vi "Logging Message Loop.vi"(6 "Metadata All":T1={"Data Fields"={"operatorName"="", "project"="", "measurementType"="", "sphere"="", "spectrometer"="", "powerSource"="", "analyzer"="", "fixtureType"="", "lampType"="", "sourceType"="", "testOrientation"="", "model"="", "sample"="", "hours"=".csv", "Amp Gain Range"=""}, "Metadata Disable"={"spectrometer"=enum."Disabled and Grayed Out", "sphere"=enum."Disabled and Grayed Out", "analyzer"=enum."Disabled and Grayed Out", "ampGainRange"=enum."Disabled and Grayed Out"}, "Output Path"=path "C:/Users/dhstuart/Dropbox/CLTC/YokogawaPZ4000/Output"}, 8 "error in (no error)":errorcluster, 9 "Stand alone?":bool=TRUE, 10 "Data Queue":refnum<queue>, 11 "Message Queues":T4) -> (0 "error out":errorcluster)   [LabVIEW 2013, in "Cal Inst Logging.lvlib"]
doc: "The message loop subVI to handle messages pertaining to logging data."
uses:
  Cal Inst Logging.lvlib
  support/Message Queue/All Message Queues.ctl
  support/Message Queue/Message Cluster.ctl
  controls/electrical2.ctl
  controls/Metadata all typedef.ctl
  controls/Metadata typedef.ctl
  controls/Metadata disable typedef.ctl
  Settings/Settings.ctl
  Acquisition/Hardware Configuration.ctl
  Logging Configuration.ctl
  Logging State.ctl
  <vilib>/Utility/error.llb/Error Cluster From Error Code.vi
  <vilib>/ErrorRing/Error Ring.xnode
  support/Message Queue/Cal Inst Message Queue.lvlib
  Acquisition/Cal Inst Acquisition.lvlib
  Settings/Cal Inst Settings.lvlib
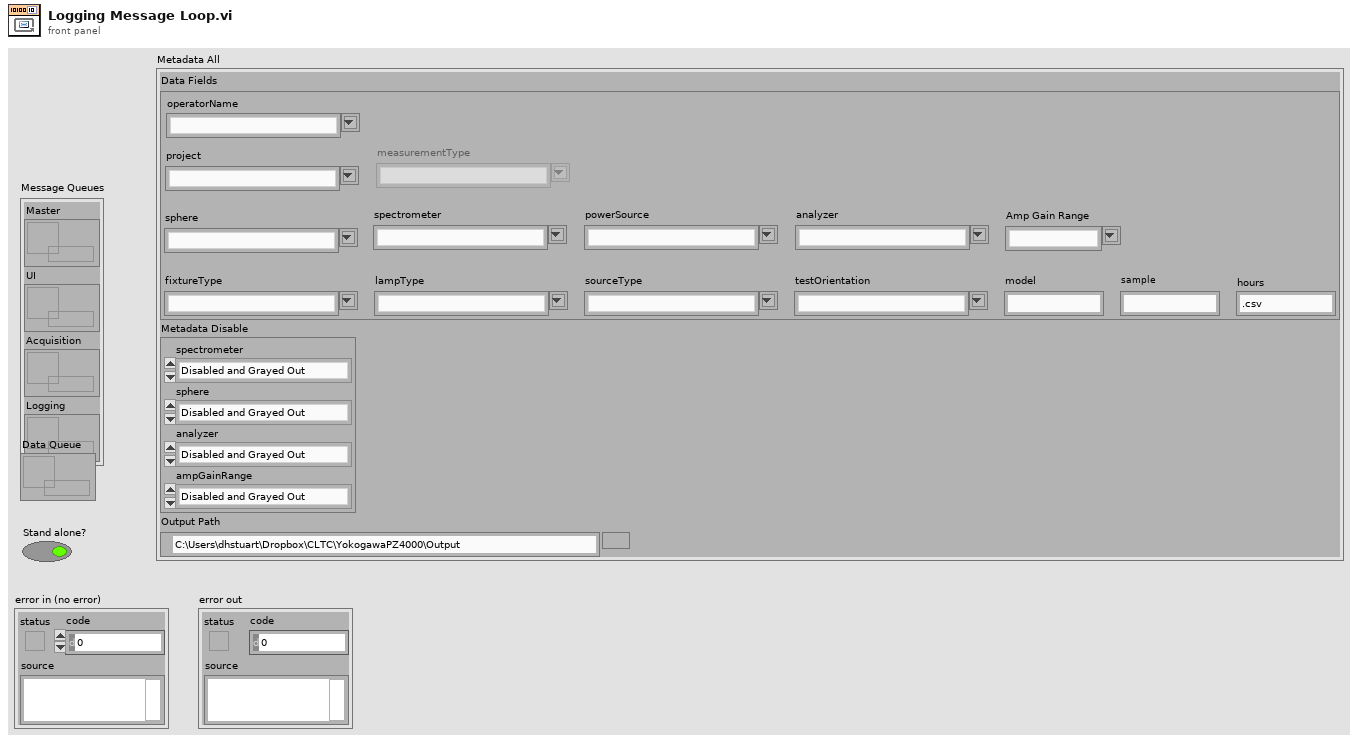
[diagram p1: front panel]
types:
  T1 = typedef "Cal Inst Logging.lvlib/Metadata all typedef.ctl" = cluster{"Data Fields":T2, "Metadata Disable":T3, "Output Path":path}
  T2 = typedef "Cal Inst Logging.lvlib/Metadata typedef.ctl" = cluster{"operatorName":string, "project":string, "measurementType":string, "sphere":string, "spectrometer":string, "powerSource":string, "analyzer":string, "fixtureType":string, "lampType":string, "sourceType":string, "testOrientation":string, "model":string, "sample":string, "hours":string, "Amp Gain Range":string}
  T3 = typedef "Cal Inst Logging.lvlib/Metadata disable typedef.ctl" = cluster{"spectrometer":enum8{"Enabled", "Disabled", "Disabled and Grayed Out"}, "sphere":enum8{"Enabled", "Disabled", "Disabled and Grayed Out"}, "analyzer":enum8{"Enabled", "Disabled", "Disabled and Grayed Out"}, "ampGainRange":enum8{"Enabled", "Disabled", "Disabled and Grayed Out"}}
  T4 = typedef "Cal Inst Message Queue.lvlib/All Message Queues.ctl" = cluster{"Master":refnum<queue>, "UI":refnum<queue>, "Acquisition":refnum<queue>, "Logging":refnum<queue>}
  T5 = typedef "Cal Inst Settings.lvlib/Settings.ctl" = cluster{"Hardware Configuration":T6, "Logging Configuration":T7}
  T6 = typedef "Cal Inst Acquisition.lvlib/Hardware Configuration.ctl" = cluster{"VISA Refnum in":refnum<visa-resource-name>, "Serial Configuration":cluster{"Baud Rate":u32, "Flow Control":u16}, "Voltage Level (0V)":dbl, "Output Phase(s) (1-Phase)":u16, "Active Phase (1:Phase 1)":i32}
  T7 = typedef "Cal Inst Logging.lvlib/Logging Configuration.ctl" = cluster{"Log File Base Path":path, "TDMS File Reference":refnum<k34>}
  T8 = typedef "Cal Inst Logging.lvlib/Logging State.ctl" = enum16{"Idle", "Logging"}
  T9 = enum16{"open", "open or create", "create or replace", "create", "open (read-only)"}
  T10 = typedef "Cal Inst Acquisition.lvlib/electrical2.ctl" = cluster{"Time Stamp":timestamp, "Temperature (C)":dbl, "Electrical Data":string[][], "Waveform Graph":waveform(dbl)[]}
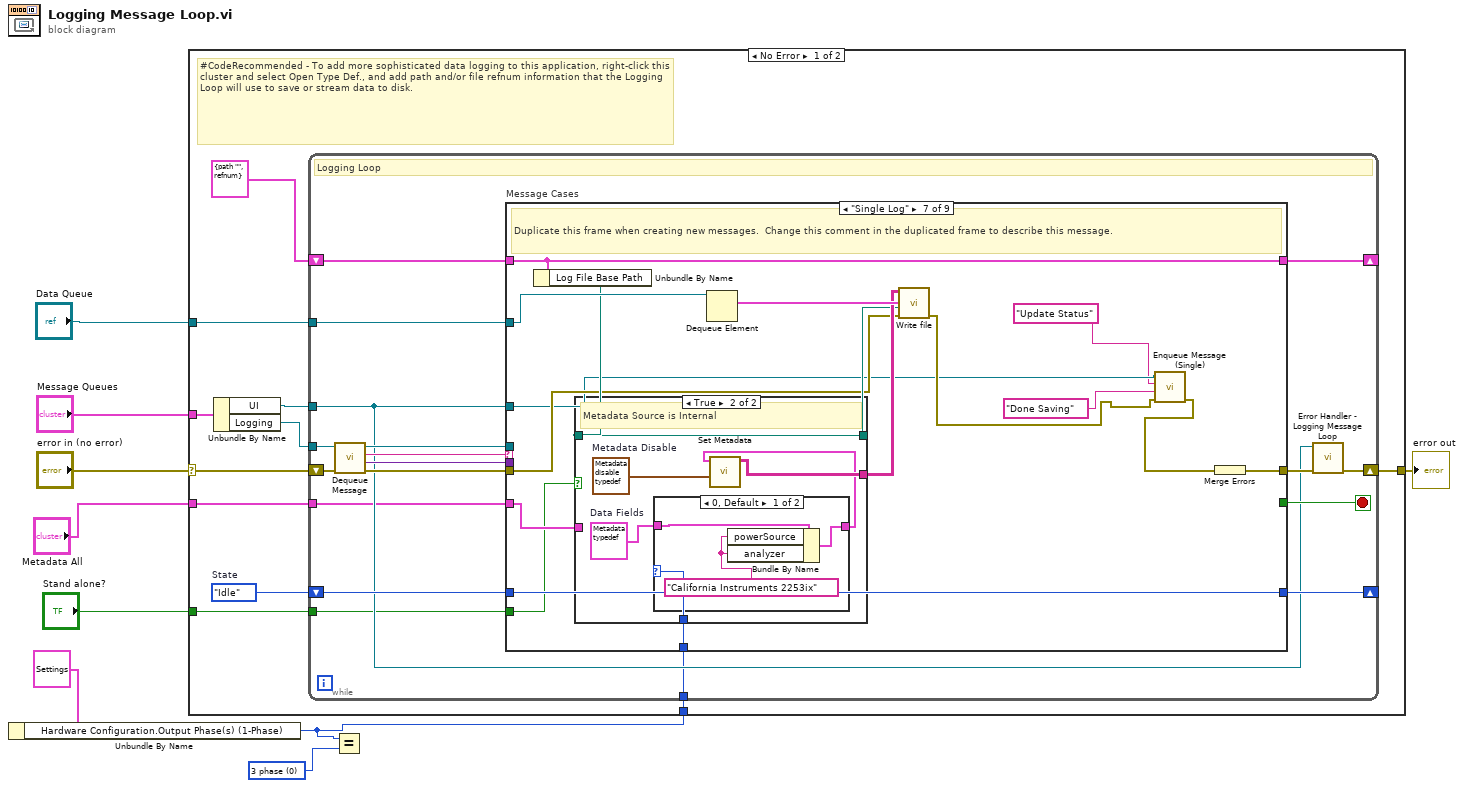
[diagram p0: block diagram]
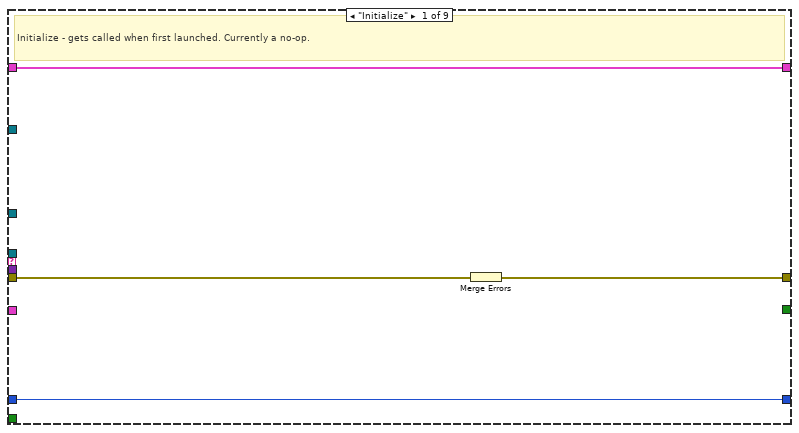
[diagram p2: hidden frame]
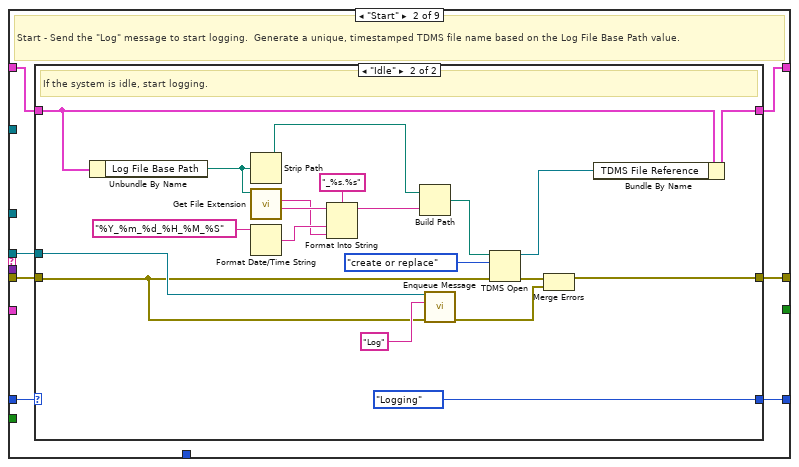
[diagram p3: hidden frame]
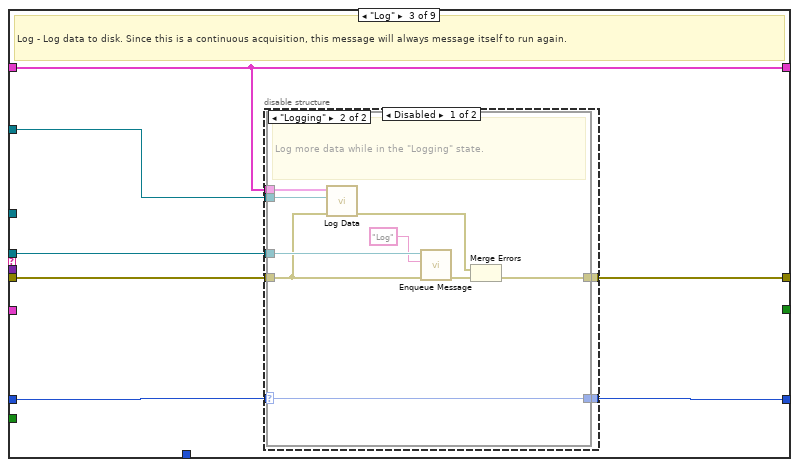
[diagram p5: hidden frame]
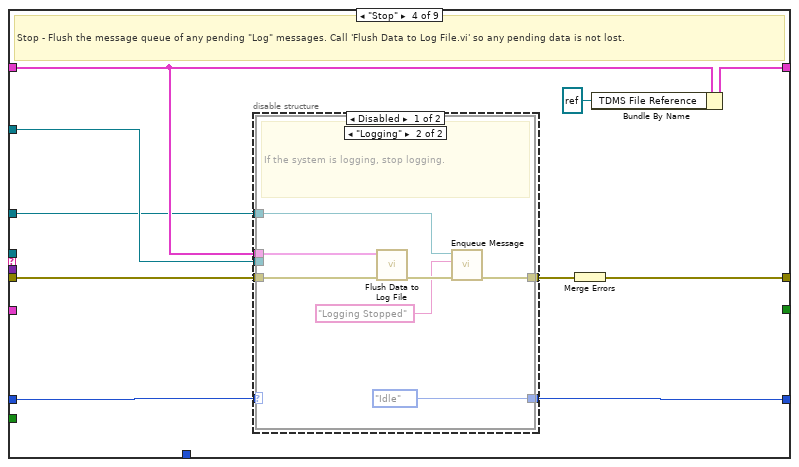
[diagram p8: hidden frame]
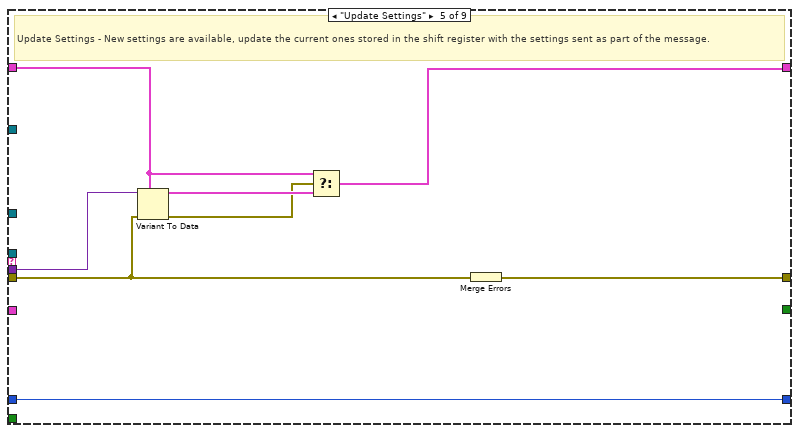
[diagram p11: hidden frame]
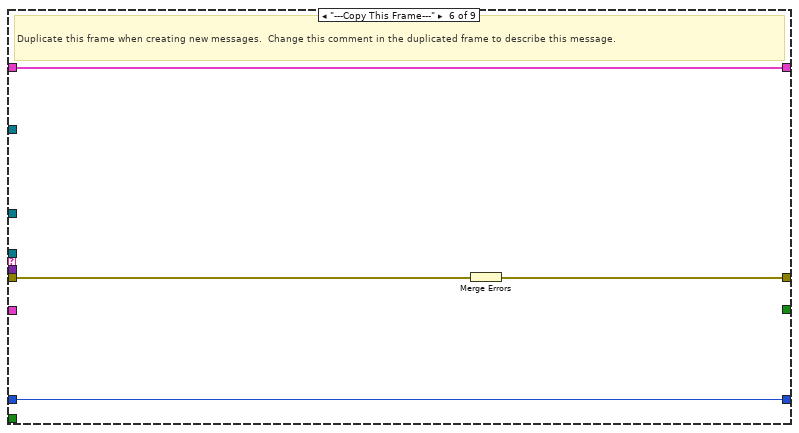
[diagram p12: hidden frame]
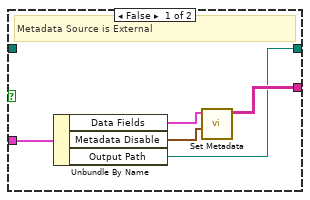
[diagram p13: hidden frame]
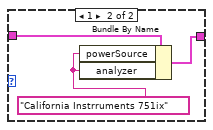
[diagram p14: hidden frame]
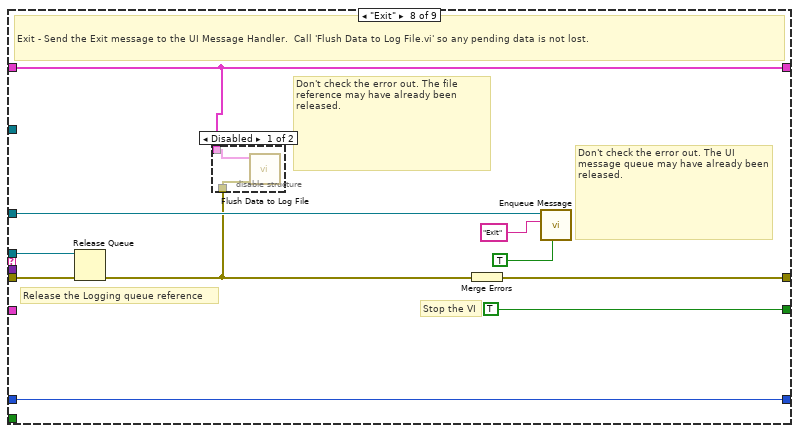
[diagram p15: hidden frame]
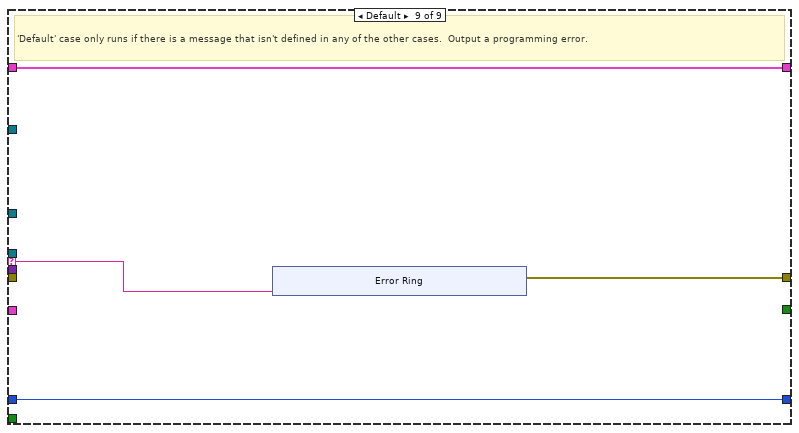
[diagram p17: hidden frame]
diagram:
  w2 = u16 0 items=["3 phase", "1 phase"] ("Output Phase(s) (1-Phase)")
  n1 = Unbundle By Name(T5 {"Hardware Configuration"={"VISA Refnum in"="", "Serial Configuration"={"Baud Rate"=0, "Flow Control"=0}, "Voltage Level (0V)"=0.0, "Output Phase(s) (1-Phase)"=0, "Active Phase (1:Phase 1)"=0}, "Logging Configuration"={"Log File Base Path"=path "", "TDMS File Reference"=refnum}} ("Settings")) -> ("Hardware Configuration.Output Phase(s) (1-Phase)"=w1:u16)
  n2 = case shown="No Error" "error in (no error)" {
    selector: "error in (no error)" -> [w16 w193]
    tunnel: "Message Queues" -> [w20 _]
    tunnel: [w18 w193] -> w8
    tunnel: "Data Queue" -> [w15 _]
    tunnel: "Metadata All" -> [w12 _]
    tunnel: "Stand alone?" -> [w11 _]
    tunnel: w1 -> [w10 _]
    frame No Error {
      w13 = Logging_State."Idle"  # State
      # "#CodeRecommended - To add more sophisticated data logging to this application, right-click this cluster and select Open Type Def., and add path and/or file refnum information that the Logging Loop will use to save or stream data to disk."
      n3 = Unbundle By Name(w20) -> ("UI"=w14:refnum<queue>, "Logging"=w19:refnum<queue>)
      n4 = while {
        tunnel: w19 -> [w30]
        shift-right: [w37] -> _
        shift-left: T7 {"Log File Base Path"=path "", "TDMS File Reference"=refnum} ("Logging Configuration") -> [w38]
        shift-right: [w26] -> w18
        shift-left: w16 -> [w35]
        tunnel: w14 -> [w24]
        tunnel: w15 -> [w29]
        shift-right: [w27] -> _
        shift-left: w13 -> [w28]
        tunnel: w12 -> [w23]
        tunnel: w11 -> [w22]
        tunnel: w10 -> [w21]
        stop <- w36 stop-if-true
        # "Logging Loop"
        n5 = call "Dequeue Message.vi"("error in (no error)"=w35, "Message Queue"=w30) -> ("error out"=w34:errorcluster, "Message Data"=w32:variant, "Message"=w33:string, "dup Message Queue"=w31:refnum<queue>)  [unwired: 6 in]
        n6 = case "Message Cases" shown="\"Single Log\"" w33 {
          selector: w33 -> [_ _ _ _ _ _ _ _ w182]
          tunnel: w31 -> [_ w48 w78 _ _ _ _ w173 _]
          tunnel: w34 -> [w40 w47 w76 w101 w125 w135 w144 w176 _]
          tunnel: [w42 w49 w79 w107 w131 w133 w152 w178 w183] -> w25
          tunnel: w38 -> [w41 w46 w75 w102 w129 w134 w147 w171 w185]
          tunnel: [w41 w45 w75 w105 w126 w134 w147 w171 w185] -> w37
          tunnel: [_ _ _ _ _ _ _ TRUE _] -> w36
          tunnel: w32 -> [_ _ _ _ w130 _ _ _ _]
          tunnel: w24 -> [_ _ _ w98 _ _ w139 w177 _]
          tunnel: w29 -> [_ _ w77 w103 _ _ w150 _ _]
          tunnel: w28 -> [w39 w44 w74 w100 w124 w132 w151 w170 w184]
          tunnel: [w39 w43 w73 w99 w124 w132 w151 w170 w184] -> w27
          tunnel: w23 -> [_ _ _ _ _ _ w143 _ _]
          tunnel: w22 -> [_ _ _ _ _ _ w142 _ _]
          tunnel: w21 -> [_ _ _ _ _ _ w136 _ _]
          frame "Initialize" {
            # "Initialize - gets called when first launched. Currently a no-op."
            n7 = Merge Errors(w40) -> (w42:errorcluster)
          }
          frame "Start" {
            # "Start - Send the \"Log\" message to start logging.  Generate a unique, timestamped TDMS file name based on the Log File Base Path value."
            n8 = case shown="\"Idle\"" w44 {
              selector: w44 -> [w51 _]
              tunnel: [w50 w54] -> w49
              tunnel: w48 -> [_ w55]
              tunnel: w47 -> [w50 w53]
              tunnel: w46 -> [w52 w56]
              tunnel: [w52 w58] -> w45
              tunnel: [w51 Logging_State."Logging" ("State")] -> w43
              frame "Logging" {
                # "The system is already logging. Ignore the \"Start\" message."
              }
              frame "Idle" {
                # "If the system is idle, start logging."
                n9 = Unbundle By Name(w56) -> ("Log File Base Path"=w71:path)
                n10 = Strip Path(path=w71) -> (stripped path=w68:path)  [unwired: 1 out]
                n11 = call <vilib>:"Get File Extension.vi"("file"=w71) -> ("filename without extension"=w69:string, "lowercase file extension"=w65:string)  [unwired: 7 in, 2 out]
                n12 = Format Date/Time String(time format string (%c)="%Y_%m_%d_%H_%M_%S") -> (date/time string=w66:string)  [unwired: 2 in]
                n13 = Format Into String(format string="_%s.%s", initial string=w69, w66, w65) -> (resulting string=w64:string)  [unwired: 1 in, 1 out]
                n14 = Build Path(base path=w68, name or relative path=w64) -> (appended path=w63:path)
                n15 = call-poly "Enqueue Message.vi"("error in (no error)"=w53, "Message"="Log", "Message Queue"=w55) -> ("error out"=w61:errorcluster)  [unwired: 7 in, 1 out]
                n16 = TDMS Open(8:w53, 10:T9."create or replace" ("operation (0:open)"), 11:w63) -> (0:w62:errorcluster, 3:w59:refnum<k34>)  [unwired: 4 in]
                n17 = Merge Errors(w62, w61) -> (w54:errorcluster)
                n18 = Bundle By Name(cluster=w56, "TDMS File Reference"=w59) -> (w58:T7)
              }
            }
          }
          frame "Log" {
            # "Log - Log data to disk. Since this is a continuous acquisition, this message will always message itself to run again."
            n19 = disable-structure shown="Disabled" {
              disable-tunnel: [w86 _] -> w79
              disable-tunnel: w78 -> [w85 _]
              disable-tunnel: w77 -> [w84 _]
              disable-tunnel: w76 -> [w83 _]
              disable-tunnel: w75 -> [w82 _]
              disable-tunnel: w74 -> [w81 _]
              disable-tunnel: [w80 _] -> w73
              frame Disabled {
                n20 = case shown="\"Logging\"" w81 {
                  selector: w81 -> [w88 w91]
                  tunnel: [w87 w97] -> w86
                  tunnel: w85 -> [_ w95]
                  tunnel: w84 -> [_ w89]
                  tunnel: w83 -> [w87 w90]
                  tunnel: w82 -> [_ w92]
                  tunnel: [w88 w91] -> w80
                  frame "Idle" {
                    # "Ignore \"Log\" messages when the logging is idle."
                  }
                  frame "Logging" {
                    # "Log more data while in the \"Logging\" state."
                    n21 = call "Log Data.vi"("error in (no error)"=w90, "Data Queue"=w89, "Logging Configuration"=w92) -> ("error out"=w94:errorcluster)  [unwired: 8 in]
                    n22 = call-poly "Enqueue Message.vi"("error in (no error)"=w90, "Message"="Log", "Message Queue"=w95) -> ("error out"=w96:errorcluster)  [unwired: 7 in, 1 out]
                    n23 = Merge Errors(w94, w96) -> (w97:errorcluster)
                  }
                }
              }
              frame Enabled {
              }
            }
          }
          frame "Stop" {
            # "Stop - Flush the message queue of any pending \"Log\" messages. Call 'Flush Data to Log File.vi' so any pending data is not lost."
            n24 = disable-structure shown="Disabled" {
              disable-tunnel: [w114 _] -> w106
              disable-tunnel: w103 -> [w113 _]
              disable-tunnel: w102 -> [w112 _]
              disable-tunnel: w101 -> [w111 _]
              disable-tunnel: w100 -> [w110 _]
              disable-tunnel: [w109 _] -> w99
              disable-tunnel: w98 -> [w108 _]
              frame Disabled {
                n25 = case shown="\"Logging\"" w110 {
                  selector: w110 -> [w115 _]
                  tunnel: [w116 w119] -> w114
                  tunnel: w113 -> [_ _]
                  tunnel: w112 -> [_ w122]
                  tunnel: w111 -> [w116 w121]
                  tunnel: [w115 Logging_State."Idle" ("State")] -> w109
                  tunnel: w108 -> [_ w118]
                  frame "Idle" {
                    # "The system is already idle. Ignore the \"Stop\" message."
                  }
                  frame "Logging" {
                    # "If the system is logging, stop logging."
                    n26 = call "Flush Data to Log File.vi"("error in (no error)"=w121, "Logging Configuration"=w122) -> ("error out"=w123:errorcluster)  [unwired: 9 in]
                    n27 = call-poly "Enqueue Message.vi"("error in (no error)"=w123, "Message"="Logging Stopped", "Message Queue"=w118) -> ("error out"=w119:errorcluster)  [unwired: 7 in, 1 out]
                  }
                }
              }
              frame Enabled {
              }
            }
            n28 = Merge Errors(w106) -> (w107:errorcluster)
            n29 = Bundle By Name(cluster=w102, "TDMS File Reference"=refnum<k34> refnum) -> (w105:T7)
          }
          frame "Update Settings" {
            # "Update Settings - New settings are available, update the current ones stored in the shift register with the settings sent as part of the message."
            n30 = Variant To Data(error in=w125, type=w129, Variant=w130) -> (data=w128:T7, error out=w127:errorcluster)
            n31 = Select(t=w129, s=w127, f=w128) -> (s? t:f=w126:T7)
            n32 = Merge Errors(w125) -> (w131:errorcluster)
          }
          frame "---Copy This Frame---" {
            # "Duplicate this frame when creating new messages.  Change this comment in the duplicated frame to describe this message."
            n33 = Merge Errors(w135) -> (w133:errorcluster)
          }
          frame "Single Log" {
            # "Duplicate this frame when creating new messages.  Change this comment in the duplicated frame to describe this message."
            n34 = Unbundle By Name(w147) -> ("Log File Base Path"=w146:path)
            n35 = case shown="True" w142 {
              tunnel: [w157 w163] -> w148
              tunnel: [w156 w162] -> w145
              tunnel: w146 -> [_ w162]
              tunnel: w143 -> [w155 _]
              tunnel: w136 -> [_ w159]
              frame False {
                # "Metadata Source is External"
                n36 = Unbundle By Name(w155) -> ("Data Fields"=w153:T2, "Metadata Disable"=w154:T3, "Output Path"=w156:path)
                n37 = call "Set Metadata.vi"("Metadata Disable"=w154, "Data Fields"=w153) -> ("Metadata Out"=w157:string[][])  [unwired: 9 in]
              }
              frame True {
                w161 = T3 {"spectrometer"=enum."Disabled and Grayed Out", "sphere"=enum."Disabled and Grayed Out", "analyzer"=enum."Disabled and Grayed Out", "ampGainRange"=enum."Disabled and Grayed Out"}  # Metadata Disable
                w160 = T2 {"operatorName"="", "project"="", "measurementType"="", "sphere"="", "spectrometer"="", "powerSource"="", "analyzer"="", "fixtureType"="", "lampType"="", "sourceType"="", "testOrientation"="", "model"="", "sample"="", "hours"="", "Amp Gain Range"=""}  # Data Fields
                # "Metadata Source is Internal"
                n38 = case shown="0, Default" w159 {
                  tunnel: w160 -> [w166 w169]
                  tunnel: [w165 w167] -> w158
                  frame 0, Default {
                    w164 = "California Instruments 2253ix" ("powerSource")
                    n39 = Bundle By Name(cluster=w166, "powerSource"=w164, "analyzer"=w164) -> (w165:T2)
                  }
                  frame 1 {
                    w168 = "California Instrruments 751ix" ("powerSource")
                    n40 = Bundle By Name(cluster=w169, "powerSource"=w168, "analyzer"=w168) -> (w167:T2)
                  }
                }
                n41 = call "Set Metadata.vi"("Metadata Disable"=w161, "Data Fields"=w158) -> ("Metadata Out"=w163:string[][])  [unwired: 9 in]
              }
            }
            n42 = Dequeue Element(queue=w150) -> (element=w149:T10)  [unwired: 2 in, 3 out]
            n43 = call "Write file.vi"("error in (no error)"=w144, "Logging Path"=w145, "Electrical Data 2"=w149, "Metadata"=w148) -> ("error out"=w141:errorcluster)  [unwired: 6 in, 1 out]
            n44 = call "Enqueue Message (Single).vi"("error in (no error)"=w141, "Message Data"="Done Saving" ("Message"), "Message"="Update Status", "Message Queue"=w139) -> ("error out"=w140:errorcluster)  [unwired: 6 in, 1 out]
            n45 = Merge Errors(w140) -> (w152:errorcluster)
          }
          frame "Exit" {
            # "Don't check the error out. The file reference may have already been released."
            # "Release the Logging queue reference"
            # "Don't check the error out. The UI message queue may have already been released."
            # "Stop the VI"
            # "Exit - Send the Exit message to the UI Message Handler.  Call 'Flush Data to Log File.vi' so any pending data is not lost."
            n46 = Release Queue(queue=w173, error in (no error)=w176) -> (error out=w172:errorcluster)  [unwired: 1 in, 2 out]
            n47 = disable-structure shown="Disabled" {
              disable-tunnel: w172 -> [w181 _]
              disable-tunnel: w171 -> [w180 _]
              frame Disabled {
                n48 = call "Flush Data to Log File.vi"("error in (no error)"=w181, "Logging Configuration"=w180) -> ()  [unwired: 9 in, 1 out]
              }
              frame Enabled {
              }
            }
            n49 = Merge Errors(w172) -> (w178:errorcluster)
            n50 = call-poly "Enqueue Message.vi"("Priority Message? (F)"=TRUE, "Message"="Exit", "Message Queue"=w177) -> ()  [unwired: 7 in, 2 out]
          }
          frame Default {
            # "'Default' case only runs if there is a message that isn't defined in any of the other cases.  Output a programming error."
            n51 = xnode "Error Ring"("parameter 0"=w182) -> ("error out"=w183:errorcluster)
          }
        }
        n52 = call "Error Handler - Logging Message Loop.vi"("error in (no error)"=w25, "Message Queue"=w24) -> ("dup error in"=w26:errorcluster)  [unwired: 8 in, 1 out]
      }
    }
    frame Error {
    }
  }
  "error out" <- w8
  n53 = Equal?(x=w1, y=w2) -> ()  [unwired: 1 out]
